vi "Read execution period (ms).vi"(8 "error in":errorcluster, 11 "Asynchronous Component Configuration in":refnum<class "asynchronous execution module configuration.lvclass">) -> (0 "error out":errorcluster, 2 "execution period (ms)":i32, 3 "Asynchronous Component Configuration out":refnum<class "asynchronous execution module configuration.lvclass">)   [LabVIEW 2013, in "asynchronous execution module configuration.lvclass"]
doc: "Reads the <b>execution period</b> property which determines the maximum rate at which the stored component can be executed."
uses:
  asynchronous execution module configuration.lvclass
  asynchronous execution module configuration.lvclass/asynchronous execution module configuration.ctl
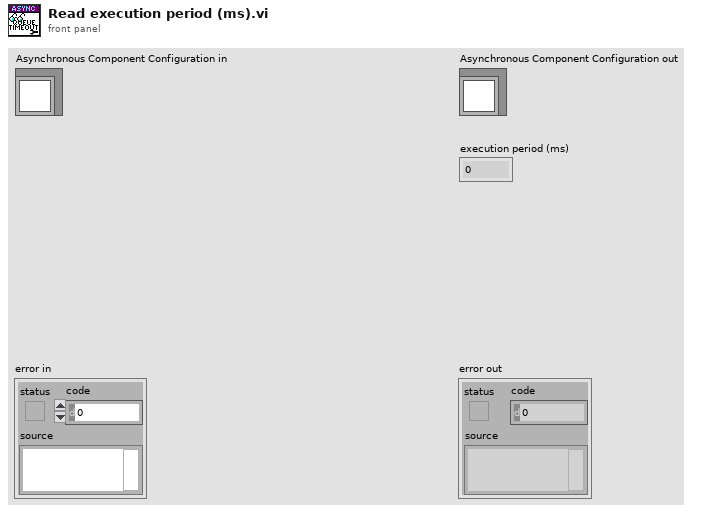
[diagram p1: front panel]
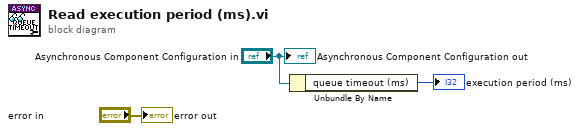
[diagram p0: block diagram]
diagram:
  n1 = Unbundle By Name("Asynchronous Component Configuration in") -> ("queue timeout (ms)"=→"execution period (ms)":i32)
  "error out" <- "error in"
  "Asynchronous Component Configuration out" <- "Asynchronous Component Configuration in"
